vi "Create.vi"(7 "Size (200)":i32=200, 8 "error in (no error)":errorcluster) -> (0 "error out":errorcluster, 3 "LocalEventCollector out":refnum<class "LocalEventCollector.lvclass">)   [LabVIEW 2020, in "Vecto.lvlib" / "LocalEventCollector.lvclass"]
uses:
  LocalEventCollector.lvclass
  LocalEventCollector.lvclass/LocalEventCollector.ctl
  lv-volatus/Volatus/Event Level.ctl
  lv-volatus/Volatus/Volatus.lvlib
  Event.ctl
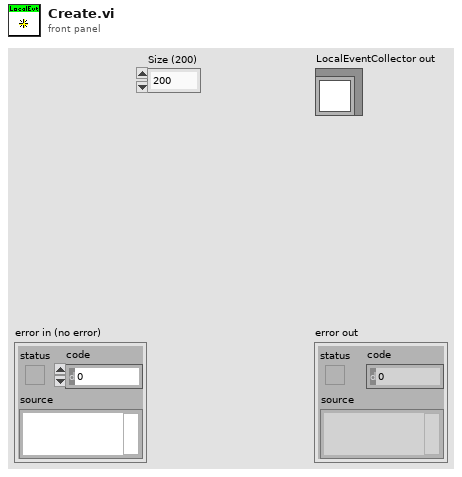
[diagram p1: front panel]
types:
  T1 = typedef "Vecto.lvlib/LocalEventCollector.lvclass/Event.ctl" = cluster{"Time Stamp":timestamp, "Event Level":T2, "Message":string, "Error":errorcluster}
  T2 = typedef "Volatus.lvlib/Event Level.ctl" = enum16{"Debug", "Info", "Warning", "Error"}
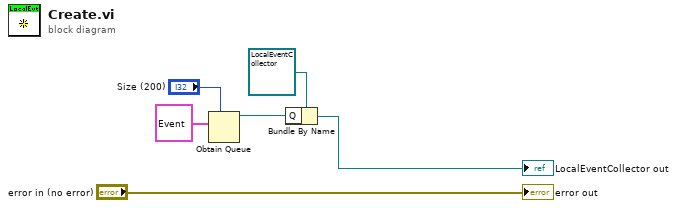
[diagram p0: block diagram]
diagram:
  n1 = Obtain Queue(max queue size (-1, unlimited)="Size (200)", element data type=T1 {"Time Stamp"=timestamp(0 s since 1904-01-01), "Event Level"=enum."Info", "Message"="", "Error"={"status"=FALSE, "code"=0, "source"=""}} ("Event")) -> (queue out=w1:refnum<queue>)  [unwired: 3 in, 2 out]
  n2 = Bundle By Name(cluster=refnum<class "LocalEventCollector.lvclass"> refnum ("LocalEventCollector in"), "Q"=w1) -> (→"LocalEventCollector out":refnum<class "LocalEventCollector.lvclass">)
  "error out" <- "error in (no error)"
